vi "Test Helper Loop.vi"(8 "error in (no error)":errorcluster, 11 "Helper Loop Test In":refnum<class "Helper Loop Test.lvclass">) -> (0 "error out":errorcluster, 3 "Helper Loop Test Out":refnum<class "Helper Loop Test.lvclass">)   [LabVIEW 2020, in "Helper Loop Test.lvclass"]
uses:
  Helper Loop Test.lvclass
  Mock Process/Mock Process.lvclass
  <vilib>/Asteme/LUnit/Test Case.lvclass
  Framework/Process/Process.lvclass
  C:/Users/anton/Documents/GitHub/Triarc-Framework/source/Framework/Process/Process.lvclass
  C:/Users/anton/Documents/GitHub/Triarc-Framework/source/Framework/Base/Base.lvclass
  C:/Users/anton/Documents/GitHub/Triarc-Framework/source/Framework/Configuration File/Configuration File.lvclass
  C:/Users/anton/Documents/GitHub/Triarc-Framework/source/Framework/Error Handler Interface/Error Handler Interface.lvclass
  C:/Users/anton/Documents/GitHub/Triarc-Framework/source/Framework Test/Mock Process/Mock Process.lvclass
  C:/Users/anton/Documents/GitHub/Triarc-Framework/source/Framework/Helper Loop/Helper Loop.lvclass
  C:/Program Files (x86)/National Instruments/LabVIEW 2020/vi.lib/Asteme/LUnit/Test Case.lvclass
  C:/Users/anton/Documents/GitHub/Triarc-Framework/source/Framework Test/Helper Loop Test/Helper Loop Test.lvclass
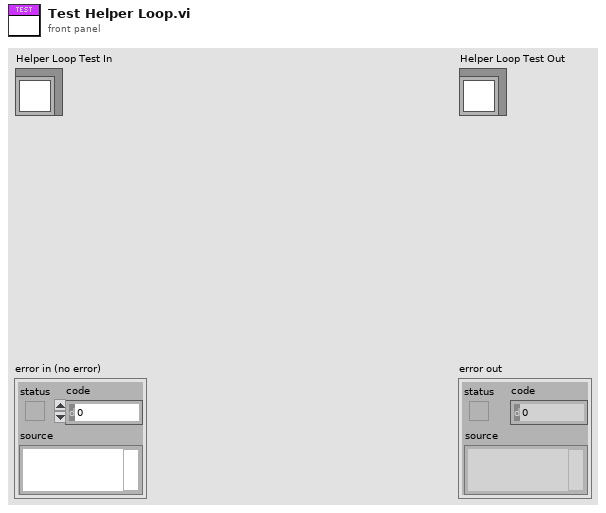
[diagram p1: front panel]
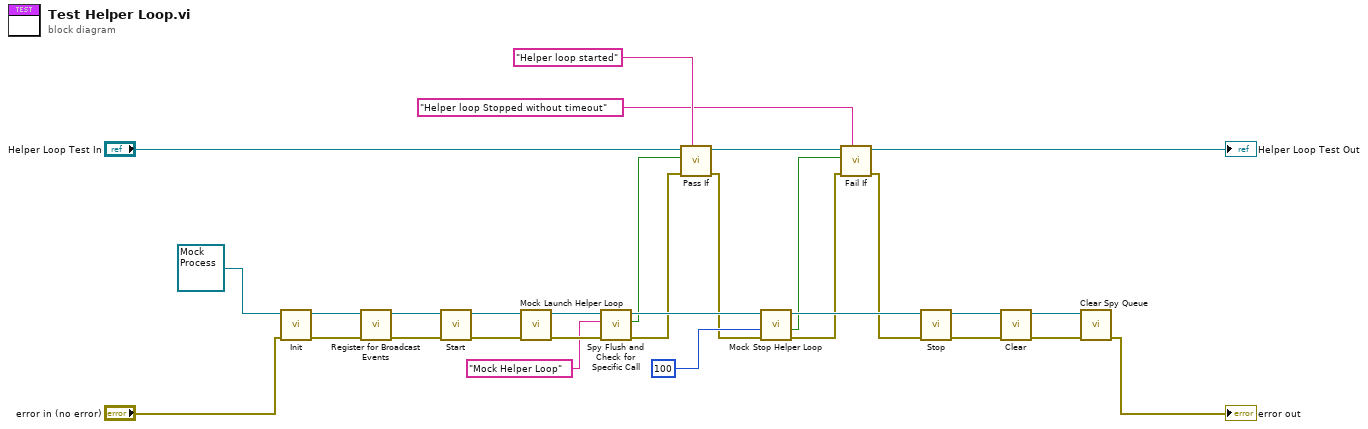
[diagram p0: block diagram]
diagram:
  n1 = call-dynamic "Init.vi"("error in (no error)"="error in (no error)", "Mock Process In"=refnum<class "Mock Process.lvclass"> refnum) -> ("error out"=w28:errorcluster, "Mock Process Out"=w29:refnum<class "Mock Process.lvclass">)  [unwired: 8 in]
  n2 = call-dynamic "Register for Broadcast Events.vi"("error in (no error)"=w28, "Process In"=w29) -> ("error out"=w26:errorcluster, "Process Out"=w27:refnum<class "Mock Process.lvclass">)  [unwired: 7 in, 1 out]
  n3 = call "Start.vi"("error in (no error)"=w26, "Process In"=w27) -> ("error out"=w24:errorcluster, "Process Out"=w25:refnum<class "Mock Process.lvclass">)  [unwired: 8 in]
  n4 = call "Mock Launch Helper Loop.vi"("error in (no error)"=w24, "Mock Process in"=w25) -> ("error out"=w13:errorcluster, "Mock Process out"=w12:refnum<class "Mock Process.lvclass">)  [unwired: 8 in]
  n5 = call "Spy Flush and Check for Specific Call.vi"("error in (no error)"=w13, "Specific Call"="Mock Helper Loop" ("Message"), "Mock Rig Process In"=w12) -> ("error out"=w7:errorcluster, "Occured?"=w5:bool, "Mock Rig Process Out"=w11:refnum<class "Mock Process.lvclass">)  [unwired: 6 in]
  n6 = call <vilib>:"Pass If.vi"("Description"="Helper loop started", "error in (no error)"=w7, "Pass?"=w5, "Test Case In"="Helper Loop Test In") -> ("error out"=w6:errorcluster, "Test Case Out"=w18:refnum<class "Helper Loop Test.lvclass">)  [unwired: 6 in]
  n7 = call "Mock Stop Helper Loop.vi"("error in (no error)"=w6, "timeout in ms (-1)"=100, "Mock Process in"=w11) -> ("error out"=w2:errorcluster, "timed out?"=w4:bool, "Mock Process out"=w23:refnum<class "Mock Process.lvclass">)  [unwired: 6 in]
  n8 = call <vilib>:"Fail If.vi"("Description"="Helper loop Stopped without timeout", "error in (no error)"=w2, "Fail?"=w4, "Test Case In"=w18) -> ("error out"=w1:errorcluster, "Test Case Out"=→"Helper Loop Test Out":refnum<class "Helper Loop Test.lvclass">)  [unwired: 6 in]
  n9 = call "Stop.vi"("error in (no error)"=w1, "Process In"=w23) -> ("error out"=w21:errorcluster, "Process Out"=w22:refnum<class "Mock Process.lvclass">)  [unwired: 7 in, 1 out]
  n10 = call-dynamic "Clear.vi"("error in (no error)"=w21, "Mock Process In"=w22) -> ("error out"=w19:errorcluster, "Mock Process Out"=w20:refnum<class "Mock Process.lvclass">)  [unwired: 8 in]
  n11 = call-dynamic "Clear Spy Queue.vi"("error in (no error)"=w19, "Mock Process In"=w20) -> ("error out"=→"error out":errorcluster)  [unwired: 8 in, 1 out]
